vi "PathPlanner_GridPosition_Get.vi"(11 "GridPosition":T1) -> (1 "Int Y":i32, 3 "Int X":i32)   [LabVIEW 2019, in "PathPlanner24.lvlib"]
uses:
  PathPlanner24.lvlib
  TypeDef/PathPlannerFinderGridPosition.ctl
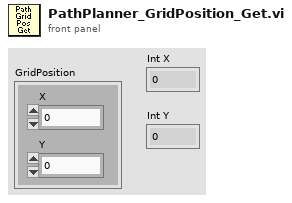
[diagram p1: front panel]
types:
  T1 = typedef "PathPlanner24.lvlib/PathPlannerFinderGridPosition.ctl" = cluster{"X":i32, "Y":i32}
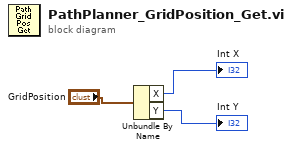
[diagram p0: block diagram]
diagram:
  n1 = Unbundle By Name("GridPosition") -> ("X"=→"Int X":i32, "Y"=→"Int Y":i32)
